vi "PowSpec.vi"() -> ()   [LabVIEW 2022 SP3]
uses:
  <vilib>/Utility/file.llb/Write To Spreadsheet File (DBL).vi
panel:
  in  "Case Constant\n(See Context Help)":bool
  out "L":dbl format="%.2f"
  out "Array":sgl[](array[numeric]) format="%.2f"
  in  "rad micros":T1={"start rad"=1.0, "step size"=1.0, "num step"=10} {"start rad" format="%.2f"; "step size" format="%.2f"}
  out "XY Graph":cluster{sgl[], dbl[]}[](graph)
  in  "con":dbl=1.0 format="%.2f"
  in  "Data System params":T2={"sample freq (MHz)"=0.0, "focal length (mm)"=50.8, "aperature radius (mm)"=4.5, "pts in window"=64.0} {"pts in window" format="%.2f"; "aperature radius (mm)" format="%.2f"; "focal length (mm)" format="%.2f"; "sample freq (MHz)" format="%.2f"}
  in  "material props":T3={"sound speed mm/micros"=1.54, "particle Z"=2.0, "host Zo"=1.0, "scatterer"=0} {"scatterer" items=["isotropic", "cylindrical", "planar"]; "host Zo" format="%.2f"; "particle Z" format="%.2f"; "sound speed mm/micros" format="%.2f"}
  in  "Tranducer Info":T4 {"bandwidth" format="%.2f"; "center freq" format="%.2f"; "start freq" format="%.2f"}
  # "Gate length"
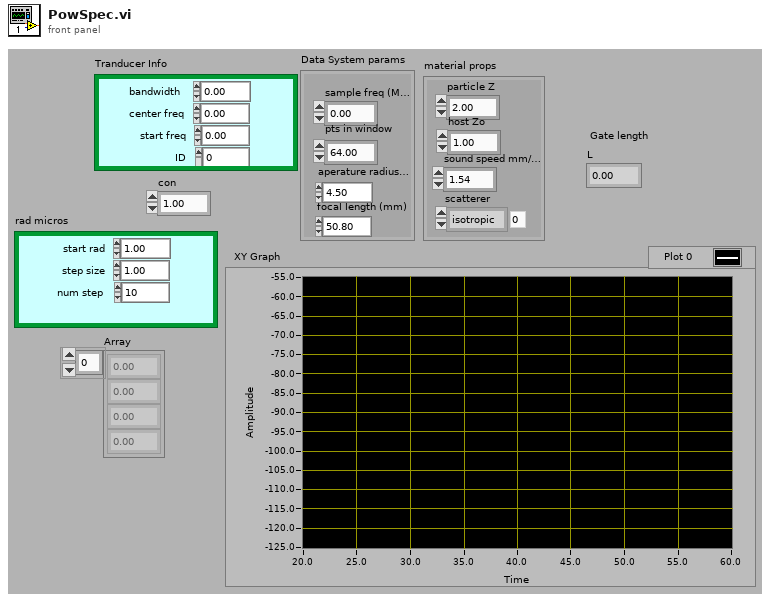
[diagram p1: front panel]
types:
  T1 = cluster{"start rad":sgl, "step size":sgl, "num step":i32}
  T2 = cluster{"sample freq (MHz)":dbl, "focal length (mm)":sgl, "aperature radius (mm)":sgl, "pts in window":dbl}
  T3 = cluster{"sound speed mm/micros":dbl, "particle Z":dbl, "host Zo":dbl, "scatterer":i32}
  T4 = cluster{"bandwidth":sgl, "center freq":sgl, "start freq":sgl, "ID":i32}
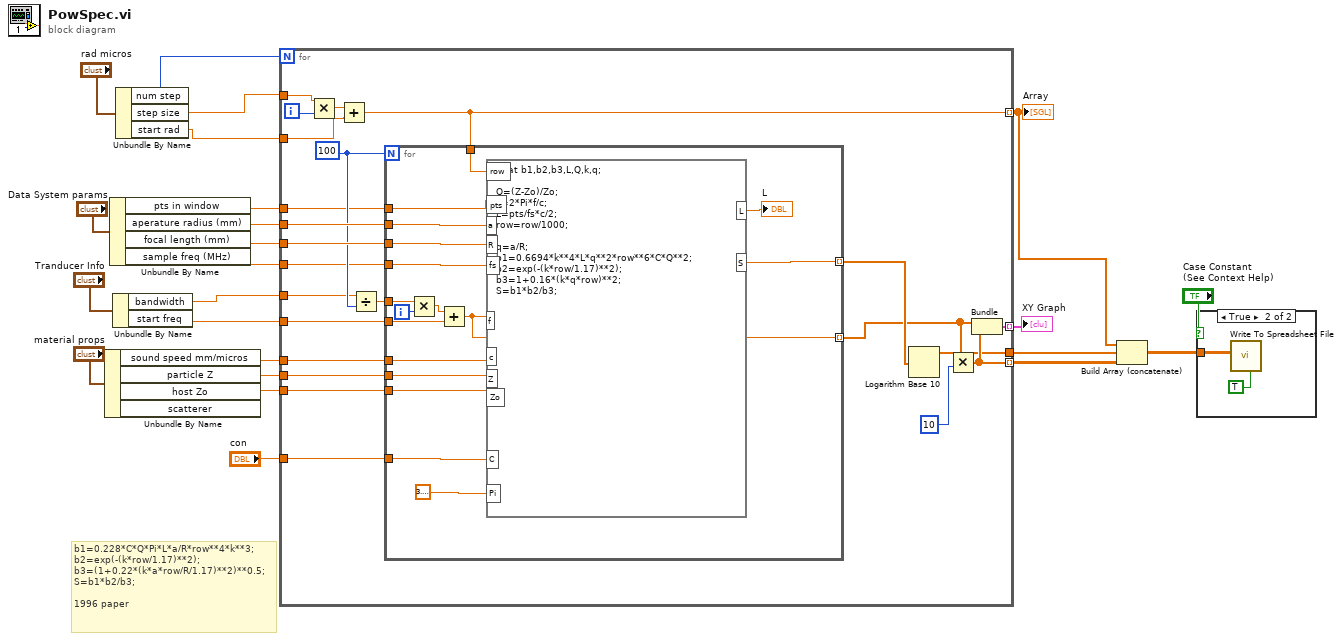
[diagram p0: block diagram]
diagram:
  # "b1=0.228*C*Q*Pi*L*a/R*row**4*k**3;\nb2=exp(-(k*row/1.17)**2);\nb3=(1+0.22*(k*a*row/R/1.17)**2)**0.5;\nS=b1*b2/b3;\n\n1996 paper"
  n1 = Unbundle By Name("material props") -> ("sound speed mm/micros"=w14:dbl, "particle Z"=w22:dbl, "host Zo"=w21:dbl)  [unwired: 1 out]
  n2 = Unbundle By Name("Data System params") -> ("pts in window"=w12:dbl, "aperature radius (mm)"=w19:sgl, "focal length (mm)"=w18:sgl, "sample freq (MHz)"=w6:dbl)
  n3 = Unbundle By Name("Tranducer Info") -> ("bandwidth"=w13:sgl, "start freq"=w15:sgl)
  n4 = Unbundle By Name("rad micros") -> ("num step"=w8:i32, "step size"=w7:sgl, "start rad"=w9:sgl)
  n5 = for {
    N: w8 -> [_]
    tunnel: w22 -> [w46]
    tunnel: w21 -> [w45]
    tunnel: w19 -> [w44]
    tunnel: w18 -> [w43]
    tunnel: "con" -> [w42]
    tunnel: w15 -> [w41]
    tunnel: w14 -> [w38]
    tunnel: w13 -> [w37]
    tunnel: w12 -> [w36]
    tunnel: [w35] -> w11 mode=indexing
    tunnel: w9 -> [w29]
    tunnel: w7 -> [w28]
    tunnel: [w27] -> w3 mode=indexing
    tunnel: w6 -> [w26]
    tunnel: [w25] -> w5 mode=indexing
    tunnel: [w24] -> w4
    i -> [w30]
    w39 = 100
    n6 = Multiply(x=w28, y=w30) -> (x*y=w31:sgl)
    n7 = Add(x=w31, y=w29) -> (x+y=w27:sgl)
    n8 = Divide(x=w37, y=w39) -> (x/y=w40:sgl)
    n9 = for {
      N: w39 -> [_]
      tunnel: w46 -> [w63]
      tunnel: w45 -> [w62]
      tunnel: w44 -> [w60]
      tunnel: w43 -> [w59]
      tunnel: w42 -> [w58]
      tunnel: [w57] -> w34 mode=indexing
      tunnel: w41 -> [w55]
      tunnel: w40 -> [w53]
      tunnel: w27 -> [w52]
      tunnel: w38 -> [w51]
      tunnel: w36 -> [w50]
      tunnel: [w49] -> w24 mode=indexing
      tunnel: w26 -> [w48]
      i -> [w56]
      n10 = Multiply(x=w53, y=w56) -> (x*y=w54:sgl)
      n11 = Add(x=w54, y=w55) -> (x+y=w49:sgl)
      n12 = formula code="float b1,b2,b3,L,Q,k,q;\n\nQ=(Z-Zo)/Zo;\nk=2*Pi*f/c;\nL=pts/fs*c/2;\nrow=row/1000;\n\nq=a/R;\nb1=0.6694*k**4*L*q**2*row**6*C*Q**2;\nb2=exp(-(k*row/1.17)**2);\nb3=1+0.16*(k*q*row)**2;\nS=b1*b2/b3;"("Z"=w63, "Zo"=w62, "Pi"=3.141592653589793, "f"=w49, "C"=w58, "row"=w52, "a"=w60, "R"=w59, "c"=w51, "fs"=w48, "pts"=w50) -> ("S"=w57:dbl, "L"=→"L":dbl)
    }
    n13 = Logarithm Base 10(1:w34) -> (0:w33:dbl[])
    n14 = Multiply(x=w33, y=10) -> (x*y=w25:dbl[])
    n15 = Bundle(w24, w25) -> (w35:cluster{sgl[], dbl[]})  [unwired: 1 out]
  }
  "XY Graph" <- w11
  "Array" <- w3
  n16 = Build Array (concatenate)(w3, w4, w5) -> (w1:dbl[][])
  n17 = case shown="True" "Case Constant\n(See Context Help)" {
    tunnel: w1 -> [_ w65]
    frame False {
    }
    frame True {
      n18 = call-poly <vilib>:"Write To Spreadsheet File.vi"("transpose? (no:F)"=TRUE, "2D data"=w65) -> ()  [unwired: 4 in, 3 out]
    }
  }
